vi "EnqueueAutoMode.vi"(6 "Priority Message":bool, 8 "error in (no error)":errorcluster, 9 "Data":variant, 10 "AutoState":T1, 11 "Queue in":refnum<queue>) -> (0 "error out":errorcluster, 3 "queue out":refnum<queue>)   [LabVIEW 2019, in "AutoMode.lvlib"]
uses:
  AutoMode.lvlib
  Enum - AutoModeState.ctl
  Cluster - AutoModeMessage.ctl
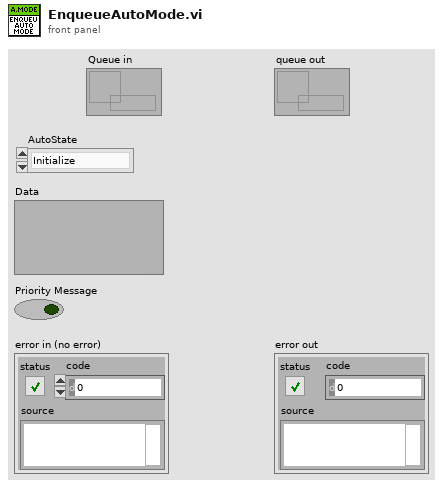
[diagram p1: front panel]
types:
  T1 = typedef "AutoMode.lvlib/Enum - AutoModeState.ctl" = enum16{"Initialize", "Idle", "UpdateConfig", "BroadcastSettings", "Start", "Winding", "WaitForWinding", "Unwind", "WaitForUnwind", "Stop", "Abort", "WriteDataToFile", "EventTriggered", "GenerateFilePath", "ZeroPosition", "GotoZero", "Error", "Exit"}
  T2 = typedef "AutoMode.lvlib/Cluster - AutoModeMessage.ctl" = cluster{"Message":T1, "Data":variant}
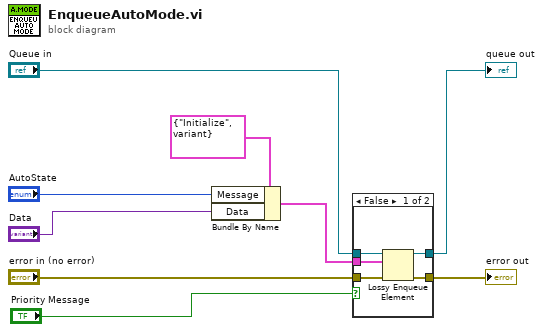
[diagram p0: block diagram]
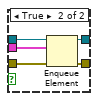
[diagram p2: hidden frame]
diagram:
  n1 = Bundle By Name(cluster=T2 {"Message"=enum."Initialize", "Data"=variant} ("CycleTestMessage"), "Message"="AutoState", "Data"="Data") -> (w7:T2)
  n2 = case shown="False" "Priority Message" {
    tunnel: [w13 w19] -> w9
    tunnel: w7 -> [w10 w18]
    tunnel: "error in (no error)" -> [w14 w17]
    tunnel: "Queue in" -> [w12 w16]
    tunnel: [w11 w15] -> w2
    frame False {
      n3 = Lossy Enqueue Element(queue=w12, element=w10, error in (no error)=w14) -> (queue out=w11:refnum<queue>, error out=w13:errorcluster)  [unwired: 2 out]
    }
    frame True {
      n4 = Enqueue Element(queue=w16, element=w18, error in (no error)=w17) -> (queue out=w15:refnum<queue>, error out=w19:errorcluster)  [unwired: 1 in, 1 out]
    }
  }
  "error out" <- w9
  "queue out" <- w2
